vi "translate error code.vi"(8 "error in (no error)":errorcluster, 10 "error code":u32 format="%x") -> (0 "error out":errorcluster)   [LabVIEW 2024, in "atsj peakcan basic.lvlib"]
doc: "Converts an <b>error code</b> into an error cluster and merges it with the <b>error in</b> cluster."
uses:
  atsj peakcan basic.lvlib
  support/x64/PCANBasic.dll
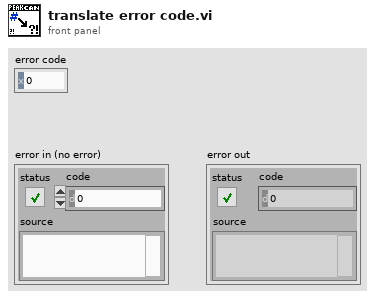
[diagram p1: front panel]
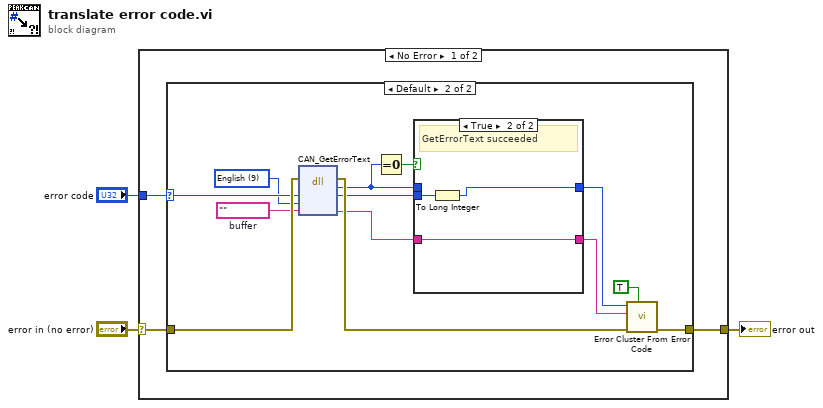
[diagram p0: block diagram]
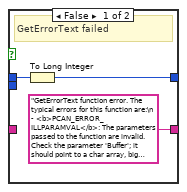
[diagram p3: hidden frame]
diagram:
  n1 = case shown="No Error" "error in (no error)" {
    selector: "error in (no error)" -> [w4 w27]
    tunnel: "error code" -> [w6 _]
    tunnel: [w5 w27] -> w1
    frame No Error {
      n2 = case shown="Default" w6 {
        selector: w6 -> [_ w19]
        tunnel: [w7 w10] -> w5
        tunnel: w4 -> [w7 w20]
        frame 0 {
        }
        frame Default {
          w16 = ""  # buffer
          w17 = u16 9 items=["System"=0, "German"=7, "English"=9, "Spanish"=10, "French"=12, "Italian"=16]
          n3 = dll-call lib="C:/atsj/plateau/atsj-peakcan-basic-for-labview/src/support/x64/PCANBasic.dll" fn="CAN_GetErrorText" label="GetErrorText"(error in=w20, "Error"=w19, "Language"=w17, "Buffer"=w16) -> (error out=w18:errorcluster, "return type"=w8:u32, "Error"=w14:u32, "Buffer"=w12:string)  [unwired: 3 in, 1 out]
          n4 = Equal To 0?(x=w8) -> (x = 0?=w15:bool)
          n5 = case shown="True" w15 {
            tunnel: w14 -> [_ w26]
            tunnel: ["GetErrorText function error. The typical errors for this function are:\n   - <b>PCAN_ERROR_ILLPARAMVAL</b>: The parameters passed to the function are invalid. Check the parameter 'Buffer'; it should point to a char array, big enough to allocate the text for the given error code.\n   - <b>PCAN_ERROR_ILLHANDLE</b>: The desired PCAN Channel is not valid. Check the list of valid Channels.\n   - <b>Invalid error code</b>: Check if the bitwise combination is correct." w25] -> w13
            tunnel: w12 -> [_ w25]
            tunnel: [w23 w24] -> w11
            tunnel: w8 -> [w21 _]
            frame False {
              # "GetErrorText failed"
              n6 = To Long Integer(number=w21) -> (32bit integer=w23:i32)
            }
            frame True {
              # "GetErrorText succeeded"
              n7 = To Long Integer(number=w26) -> (32bit integer=w24:i32)
            }
          }
          n8 = call <vilib>:"Error Cluster From Error Code.vi"("show call chain? (False)"=TRUE, "error in (no error)"=w18, "error message (\"\")"=w13, "error code (0)"=w11) -> ("error out"=w10:errorcluster)  [unwired: 5 in]
        }
      }
    }
    frame Error {
    }
  }
  "error out" <- w1
